vi "Rewire Case structure.vi"(8 "error in (no error)":errorcluster, 9 "Wire All Cases Except this One ?":i32=-1, 10 "Selector Type":variant, 11 "CaseSel Refnum":refnum<vi>) -> (0 "error out":errorcluster, 3 "CaseSel Refnum Out":refnum<vi>)   [LabVIEW 2018, in "Scripting Tools.lvlib"]
doc: "Takes a case structure and finds the first incoming tunell that has a type that matchesthe selector type variant. If the wire all cases except this one ? is set > 0 then it will wire the selector terminal to the first output terminal of the same type for all cases except the one indicated. This is mainly useful for wiring error case structures up where this control should be 1 (for the no error case)"
uses:
  Scripting Tools.lvlib
  <vilib>/Utility/VariantDataType/Type.ctl
  <vilib>/Utility/VariantDataType/VariantType.lvlib
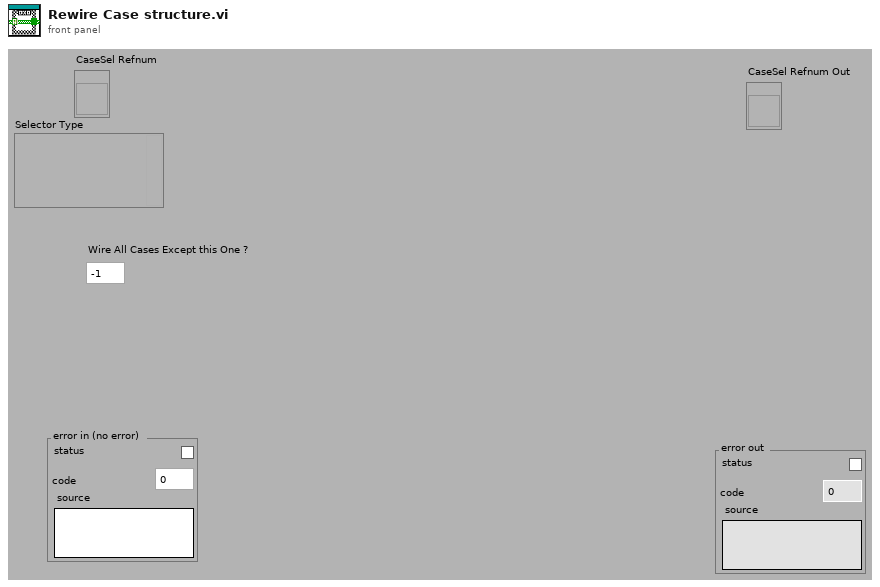
[diagram p1: front panel]
types:
  T1 = typedef "VariantType.lvlib/Type.ctl" = enum8{"Invalid Type", "Void", "I8", "I16", "I32", "I64", "U8", "U16", "U32", "U64", "Single Float", "Double Float", "Extended Float", "Single Complex", "Double Complex", "Extended Complex", "Enum U8", "Enum U16", "Enum U32", "Enum U64", "Single Float With Unit", "Double Float With Unit", "Extended Float With Unit", "Single Complex with Unit", "Double Complex with Unit", "Extended Complex with Unit", "Boolean", "String", "Path", "Picture", "Tag", "Array", "Cluster", "Variant", "LV Variant", "Waveform", "Timestamp", "Digital Waveform", "Digital Data", "ExpressData", "Refnum", "External Data", "VI", "Poly VI", "LabVIEW Class Instance", "Fixed Point"}
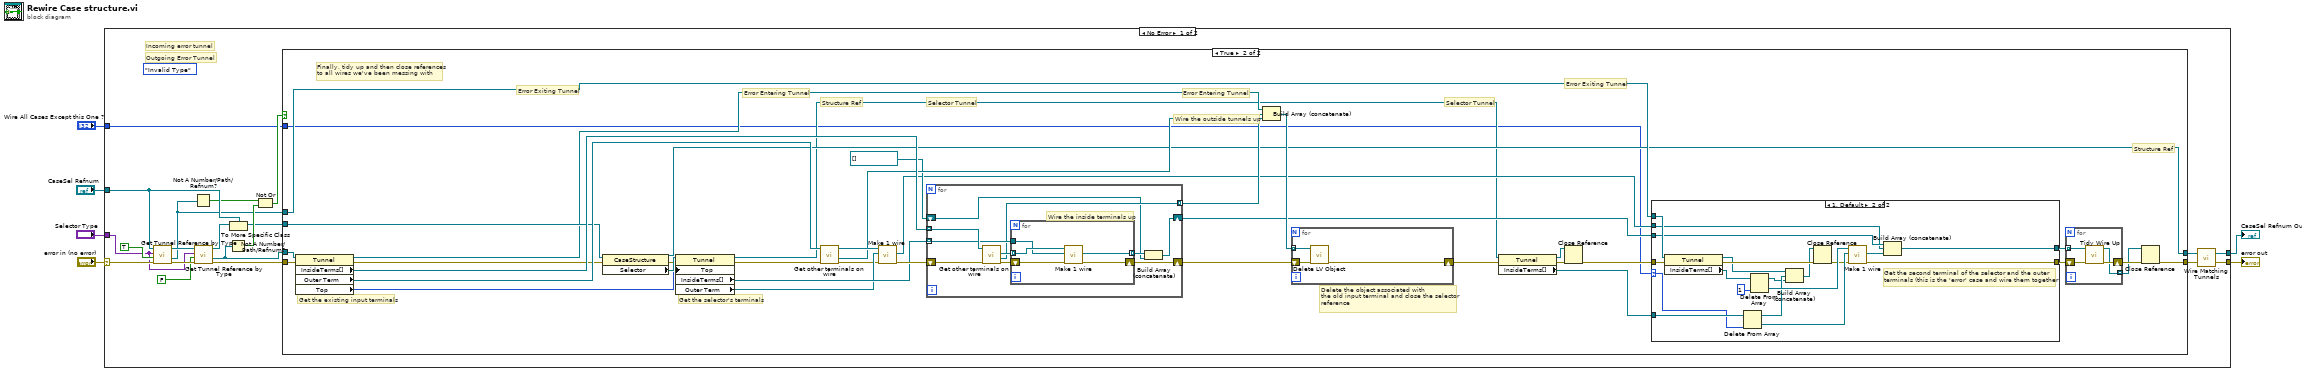
[diagram p0: block diagram]
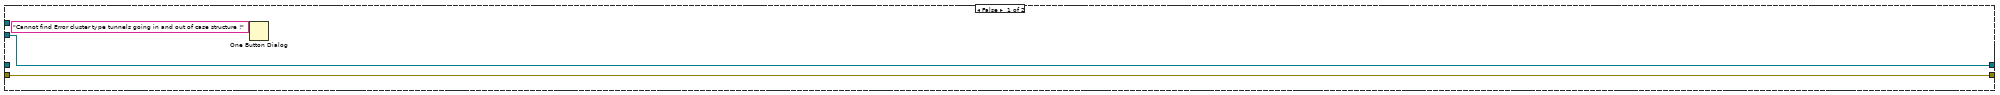
[diagram p2: hidden frame]
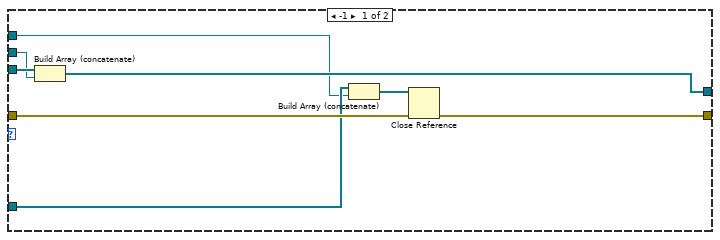
[diagram p3: hidden frame]
diagram:
  n1 = case shown="No Error" "error in (no error)" {
    selector: "error in (no error)" -> [w12 w117]
    tunnel: "CaseSel Refnum" -> [w25 w116]
    tunnel: [w9 w116] -> w4
    tunnel: [w7 w117] -> w1
    tunnel: "Selector Type" -> [w11 _]
    tunnel: "Wire All Cases Except this One ?" -> [w10 _]
    frame No Error {
      (unwired) Type."Invalid Type" ("Type Enum")
      # "Outgoing Error Tunnel"
      # "Incoming error tunnel"
      n2 = call "Get Tunnel Reference by Type.vi"("error IO"=w12, "Input Tunnel (F)/Output Tunnel (T)"=TRUE, "Tunnel Type"=w11, "Case Refnum In"=w25) -> ("error out"=w24:errorcluster, "Desired Tunnel Reference"=w17:refnum<vi>, "Case Refnum Out"=w23:refnum<vi>)  [unwired: 5 out]
      n3 = Not A Number/Path/Refnum?(number/path/refnum=w17) -> (NaN/Path/Refnum?=w18:bool)
      n4 = call "Get Tunnel Reference by Type.vi"("error IO"=w24, "Input Tunnel (F)/Output Tunnel (T)"=FALSE, "Tunnel Type"=w11, "Case Refnum In"=w23) -> ("error out"=w14:errorcluster, "Desired Tunnel Reference"=w16:refnum<vi>, "Case Refnum Out"=w21:refnum<vi>)  [unwired: 5 out]
      n5 = Not A Number/Path/Refnum?(number/path/refnum=w16) -> (NaN/Path/Refnum?=w19:bool)
      n6 = To More Specific Class(target class=w25, reference=w21) -> (specific class reference=w15:refnum<vi>)  [unwired: 1 in, 1 out]
      n7 = Not Or(1:w19, 2:w18) -> (0:w20:bool)
      n8 = case shown="True" w20 {
        tunnel: w14 -> [w29 w45]
        tunnel: w16 -> [_ w66]
        tunnel: w17 -> [_ w58]
        tunnel: [w29 w32] -> w8
        tunnel: w15 -> [w27 w47]
        tunnel: [w27 w42] -> w13
        tunnel: w10 -> [_ w30]
        frame False {
          n9 = One Button Dialog(message="Cannot find Error cluster type tunnels going in and out of case structure !") -> ()  [unwired: 2 out]
        }
        frame True {
          # "Finally, tidy up and then close references\nto all wires we've been messing with"
          # "Delete the object associated with \nthe old input terminal and close the selector\nreference"
          # "Selector Tunnel"
          # "Error Exiting Tunnel"
          # "Error Entering Tunnel"
          # "Structure Ref"
          # "Selector Tunnel"
          # "Structure Ref"
          # "Error Entering Tunnel"
          # "Error Exiting Tunnel"
          # "Get the selector's terminals"
          # "Get the existing input terminals"
          # "Wire the outside tunnels up"
          n10 = property class="Tunnel"(reference=w66, error in=w45) -> (reference out=w40:refnum<vi>, error out=w39:errorcluster, "InsideTerms[]"=w63:refnum<vi>[], "Outer Term"=w65:refnum<vi>, "Top"=w41:i32)
          n11 = property class="CaseStructure"(reference=w47, error in=w39) -> (reference out=w42:refnum<vi>, error out=w44:errorcluster, "Selector"=w46:refnum<vi>)
          n12 = property class="Tunnel"(reference=w46, error in=w44, "Top"=w41) -> (reference out=w35:refnum<vi>, error out=w43:errorcluster, "InsideTerms[]"=w38:refnum<vi>[], "Outer Term"=w37:refnum<vi>)
          n13 = call "Get other terminals on wire.vi"("error in (no error)"=w43, "Reference"=w65) -> ("error out"=w36:errorcluster, "Wire"=w54:refnum<vi>, "Source Terminal"=w64:refnum<vi>)  [unwired: 7 out]
          n14 = call "Make 1 wire.vi"("error in"=w36, "Wire Terminal 2"=w37, "Wire Terminal 1"=w64) -> ("error out"=w62:errorcluster, "Wire"=w48:refnum<vi>)  [unwired: 7 out]
          n15 = for {
            tunnel: w63 -> [w110] mode=indexing
            tunnel: w38 -> [w106] mode=indexing
            shift-right: [w105] -> w61
            shift-left: w62 -> [w109]
            tunnel: [w104] -> w56 mode=indexing
            shift-right: [w102] -> w52
            shift-left: refnum<vi>[] [] -> [w101]
            # "Wire the inside terminals up"
            n16 = call "Get other terminals on wire.vi"("error in (no error)"=w109, "Reference"=w110) -> ("error out"=w108:errorcluster, "Wire"=w104:refnum<vi>, "Sink Terminals"=w107:refnum<vi>[])  [unwired: 7 out]
            n17 = for {
              shift-right: [w112] -> w105
              shift-left: w108 -> [w115]
              tunnel: w107 -> [w114] mode=indexing
              tunnel: w106 -> [w113]
              tunnel: [w111] -> w103 mode=indexing
              n18 = call "Make 1 wire.vi"("error in"=w115, "Wire Terminal 2"=w113, "Wire Terminal 1"=w114) -> ("error out"=w112:errorcluster, "Wire"=w111:refnum<vi>)  [unwired: 7 out]
            }
            n19 = Build Array (concatenate)(w103, w101) -> (w102:refnum<vi>[])
          }
          n20 = Build Array (concatenate)(w40, w56, w54) -> (w55:refnum<vi>[])
          n21 = for {
            shift-right: [w99] -> w60
            shift-left: w61 -> [w100]
            tunnel: w55 -> [w98] mode=indexing
            n22 = call "Delete LV Object.vi"("error out 2"=w100, "reference"=w98) -> ("error out"=w99:errorcluster)  [unwired: 8 out]
          }
          n23 = property class="Tunnel"(reference=w35, error in=w60) -> (reference out=w33:refnum<vi>, error out=w59:errorcluster, "InsideTerms[]"=w57:refnum<vi>[])
          n24 = Close Reference(reference=w33, error in (no error)=w59) -> (error out=w34:errorcluster)
          n25 = case shown="1, Default" w30 {
            selector: w30 -> [_ w75]
            tunnel: w58 -> [w69 w93]
            tunnel: w57 -> [w70 w92]
            tunnel: w52 -> [w73 w86]
            tunnel: [w68 w85] -> w51
            tunnel: [w71 w84] -> w50
            tunnel: w48 -> [w72 w82]
            tunnel: w34 -> [w74 w79]
            frame -1 {
              n26 = Build Array (concatenate)(w73, w72) -> (w71:refnum<vi>[])
              n27 = Build Array (concatenate)(w70, w69) -> (w67:refnum<vi>[])
              n28 = Close Reference(reference=w67, error in (no error)=w74) -> (error out=w68:errorcluster)
            }
            frame 1, Default {
              # "Get the second terminal of the selector and the outer\nterminals (this is the 'error' case and wire them together"
              n29 = property class="Tunnel"(reference=w93, error in=w79) -> (reference out=w80:refnum<vi>, error out=w87:errorcluster, "InsideTerms[]"=w91:refnum<vi>[])
              n30 = Delete From Array(array=w92, index=w75) -> (deleted portion=w88:refnum<vi>, array with subset deleted=w77:refnum<vi>[])  [unwired: 1 in]
              n31 = Delete From Array(array=w91, index=1) -> (deleted portion=w89:refnum<vi>, array with subset deleted=w76:refnum<vi>[])  [unwired: 1 in]
              n32 = Build Array (concatenate)(w80, w77, w76) -> (w78:refnum<vi>[])
              n33 = Close Reference(reference=w78, error in (no error)=w87) -> (error out=w81:errorcluster)
              n34 = call "Make 1 wire.vi"("error in"=w81, "Wire Terminal 2"=w88, "Wire Terminal 1"=w89) -> ("error out"=w85:errorcluster, "Wire"=w83:refnum<vi>)  [unwired: 7 out]
              n35 = Build Array (concatenate)(w86, w82, w83) -> (w84:refnum<vi>[])
            }
          }
          n36 = for {
            shift-right: [w96] -> w49
            shift-left: w51 -> [w97]
            tunnel: w50 -> [w95] mode=indexing
            tunnel: [w94] -> w31 mode=indexing
            n37 = call "Tidy Wire Up.vi"("error in (no error)"=w97, "Wire"=w95) -> ("error out"=w96:errorcluster, "Out"=w94:refnum<vi>)  [unwired: 2 in, 6 out]
          }
          n38 = Close Reference(reference=w31, error in (no error)=w49) -> (error out=w32:errorcluster)
        }
      }
      n39 = call "Wire Matching Tunnels.vi"("Error In"=w8, "Case Refnum"=w13) -> ("error out"=w7:errorcluster, "Case Refnum"=w9:refnum<vi>)
    }
    frame Error {
    }
  }
  "CaseSel Refnum Out" <- w4
  "error out" <- w1
